vi "Delete Empty Folders.vi"(4 "dirpath":path caption="Directory Path") -> (0 "error out":errorcluster)   [LabVIEW 2017, in "File IO.lvclass"]
uses:
  File IO.lvclass
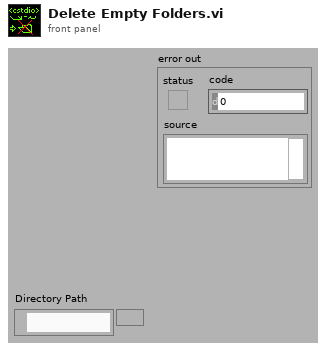
[diagram p1: front panel]
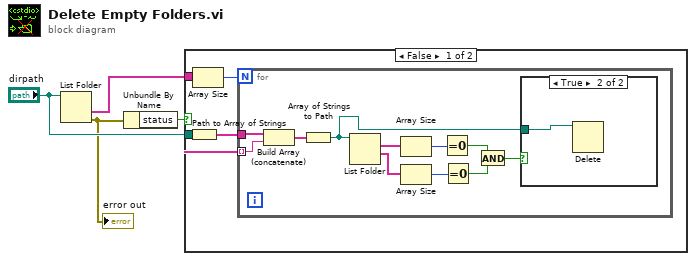
[diagram p0: block diagram]
diagram:
  n1 = List Folder(path="dirpath") -> (folder names=w4:string[], error out=w2:errorcluster)  [unwired: 1 in, 4 out]
  "error out" <- w2
  n2 = Unbundle By Name(w2) -> ("status"=w1:bool)
  n3 = case shown="False" w1 {
    tunnel: w4 -> [w7 _]
    tunnel: "dirpath" -> [w6 _]
    frame False {
      n4 = Path to Array of Strings(0:w6) -> (2:w5:string[])  [unwired: 1 out]
      n5 = Array Size(array=w7) -> (size(s)=w8:i32)
      n6 = for {
        N: w8 -> [_]
        tunnel: w7 -> [w18] mode=indexing
        tunnel: w5 -> [w19]
        n7 = Build Array (concatenate)(w19, w18) -> (w17:string[])
        n8 = Array of Strings to Path(0:w17) -> (2:w10:path)  [unwired: 1 out]
        n9 = List Folder(path=w10) -> (filenames=w16:string[], folder names=w15:string[])  [unwired: 1 in, 4 out]
        n10 = Array Size(array=w16) -> (size(s)=w14:i32)
        n11 = Array Size(array=w15) -> (size(s)=w13:i32)
        n12 = Equal To 0?(x=w14) -> (x = 0?=w12:bool)
        n13 = Equal To 0?(x=w13) -> (x = 0?=w11:bool)
        n14 = And(x=w12, y=w11) -> (x .and. y?=w9:bool)
        n15 = case shown="True" w9 {
          tunnel: w10 -> [_ w20]
          frame False {
          }
          frame True {
            n16 = Delete(path (use dialog)=w20) -> ()  [unwired: 1 in, 6 out]
          }
        }
      }
    }
    frame True {
    }
  }
